vi "MIC_X_OUT_DIAG_HIGHRES_Formula.vi"(11 "Numeric in":u32) -> (3 "Numeric out":dbl)   [LabVIEW 2015]
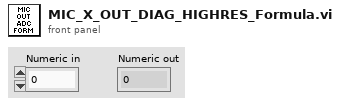
[diagram p1: front panel]
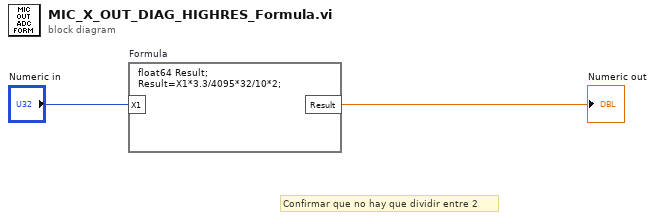
[diagram p0: block diagram]
diagram:
  # "Confirmar que no hay que dividir entre 2"
  n1 = formula code="float64 Result;\nResult=X1*3.3/4095*32/10*2;"("X1"="Numeric in") -> ("Result"=→"Numeric out":dbl)
